vi "Console Wrapper Example.vi"   [LabVIEW 2020, in "Console Wrapper.lvclass"]
uses:
  Console Wrapper.lvclass
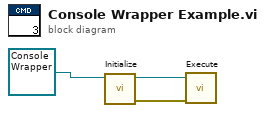
[diagram p0: block diagram]
diagram:
  n1 = call-dynamic "Initialize.vi"("Console Wrapper in"=refnum<class "Console Wrapper.lvclass"> refnum) -> ("error out"=w2:errorcluster, "Console Wrapper out"=w3:refnum<class "Console Wrapper.lvclass">)  [unwired: 9 in]
  n2 = call "Execute.vi"("error in (no error)"=w2, "Console Wrapper in"=w3) -> ()  [unwired: 7 in, 3 out]
